vi "Persistent Feature Toggle Page.vi"(5 "feature disabled vi":refnum<vi>, 7 "feature enabled vi":refnum<vi>, 8 "error in (no error)":errorcluster, 9 "Node Ptr":T1 format="%.0x", 10 "property name":string, 11 "SubPanel in":refnum<vi>) -> (0 "error out":errorcluster, 3 "SubPanel out":refnum<vi>)   [LabVIEW 2017, in "Engine Simulation Toolkit System Explorer.lvlib"]
uses:
  Engine Simulation Toolkit System Explorer.lvlib
  <vilib>/NI Veristand/Custom Device API/Custom Device Item Ref.ctl
  <vilib>/NI Veristand/Custom Device API/Get Item Property (Boolean).vi
  <vilib>/NI Veristand/Custom Device API/Custom Device API.lvlib
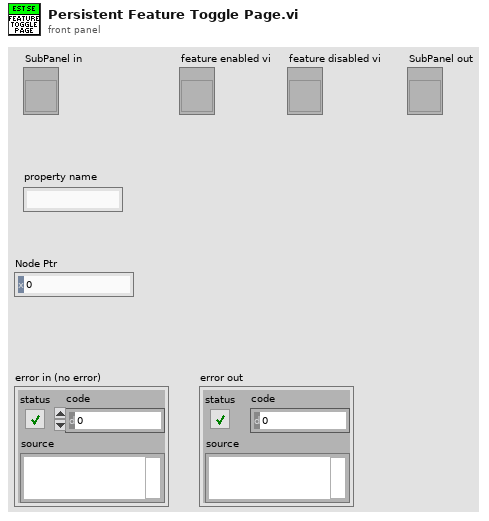
[diagram p1: front panel]
types:
  T1 = typedef "Custom Device API.lvlib/Custom Device Item Ref.ctl" = u64
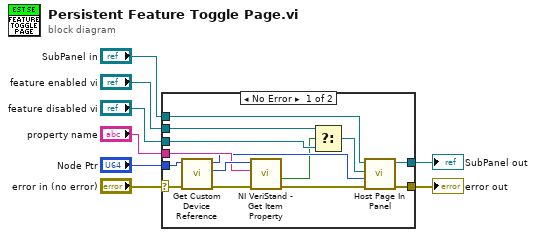
[diagram p0: block diagram]
diagram:
  n1 = case shown="No Error" "error in (no error)" {
    selector: "error in (no error)" -> [w13 w24]
    tunnel: [w22 w24] -> w7
    tunnel: "SubPanel in" -> [w21 w23]
    tunnel: "Node Ptr" -> [w14 _]
    tunnel: "feature enabled vi" -> [w20 _]
    tunnel: "feature disabled vi" -> [w19 _]
    tunnel: [w17 w23] -> w2
    tunnel: "property name" -> [w12 _]
    frame No Error {
      n2 = call "Get Custom Device Reference.vi"("error in (no error)"=w13, "Item Ref in"=w14) -> ("error out"=w15:errorcluster, "Custom Device Ref"=w16:T1, "Item Ref out"=w10:T1)  [unwired: 7 in]
      n3 = call-poly <vilib>:"NI VeriStand - Get Item Property.vi"("error in (no error)"=w15, "Property Name"=w12, "Item Ref in"=w16) -> ("error out"=w11:errorcluster, "Value"=w9:bool)  [unwired: 5 in, 2 out]
      n4 = Select(t=w20, s=w9, f=w19) -> (s? t:f=w18:refnum<vi>)
      n5 = call "Host Page In Panel.vi"("error in (no error)"=w11, "Node Ptr"=w10, "VI Refnum in"=w18, "SubPanel in"=w21) -> ("error out"=w22:errorcluster, "SubPanel out"=w17:refnum<vi>)  [unwired: 5 in, 1 out]
    }
    frame Error {
    }
  }
  "error out" <- w7
  "SubPanel out" <- w2
